vi "Component Directory Not Found.vi"(7 "error source vi name":string, 8 "error in (no error)":errorcluster, 10 "configured path":path, 11 "Component Loader in":refnum<class "Component Loader.lvclass">) -> (0 "error out":errorcluster, 3 "Component Loader out":refnum<class "Component Loader.lvclass">)   [LabVIEW 2017, in "DSF Core.lvlib" / "Component Loader.lvclass"]
uses:
  Component Loader.lvclass
  Errors.ctl
  <vilib>/NI/Memory Manager/Static Error Handling.lvlib
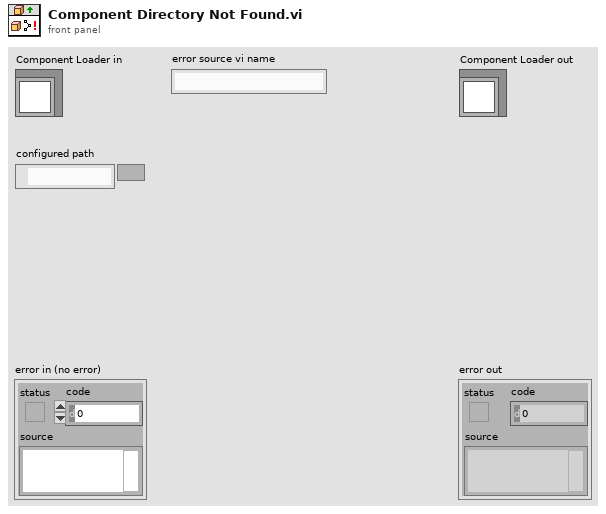
[diagram p1: front panel]
types:
  T1 = typedef "DSF Core.lvlib/Component Loader.lvclass/Errors.ctl" = enum16{"Component Directory Not Found", "Component Not Found", "Class Not Found"}
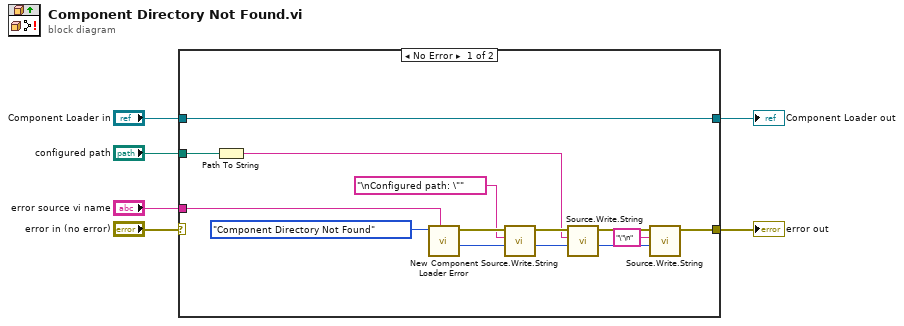
[diagram p0: block diagram]
diagram:
  n1 = case shown="No Error" "error in (no error)" {
    selector: "error in (no error)" -> [_ w22]
    tunnel: [w8 w22] -> w5
    tunnel: "error source vi name" -> [w19 _]
    tunnel: "Component Loader in" -> [w18 w21]
    tunnel: [w18 w21] -> w2
    tunnel: "configured path" -> [w17 _]
    frame No Error {
      n2 = Path To String(path=w17) -> (string=w11:string)
      n3 = call "New Component Loader Error.vi"("error source vi name"=w19, "error"=Errors."Component Directory Not Found") -> ("new offset"=w15:i32, "error out"=w16:errorcluster)  [unwired: 8 in]
      n4 = call <vilib>:"Source.Write.String.vi"("offset"=w15, "string"="\nConfigured path: \"", "error in"=w16) -> ("new offset"=w14:i32, "error out"=w13:errorcluster)  [unwired: 7 in]
      n5 = call <vilib>:"Source.Write.String.vi"("offset"=w14, "string"=w11, "error in"=w13) -> ("new offset"=w9:i32, "error out"=w10:errorcluster)  [unwired: 7 in]
      n6 = call <vilib>:"Source.Write.String.vi"("offset"=w9, "string"="\"\n", "error in"=w10) -> ("error out"=w8:errorcluster)  [unwired: 7 in, 1 out]
    }
    frame Error {
    }
  }
  "error out" <- w5
  "Component Loader out" <- w2
